vi "SetDev AFG Resource.vi"(8 "error in (no error)":errorcluster, 9 "AFG VISA Addr":refnum<visa-resource-name>, 10 "Simulated":bool, 11 "Actor_AFG in":refnum<class "Actor_AFG.lvclass">) -> (0 "error out":errorcluster, 3 "Actor_AFG out":refnum<class "Actor_AFG.lvclass">)   [LabVIEW 2020, in "Actor_AFG.lvlib" / "Actor_AFG.lvclass"]
uses:
  Actor_AFG.lvclass
  Actor_AFG.lvclass/Actor_AFG.ctl
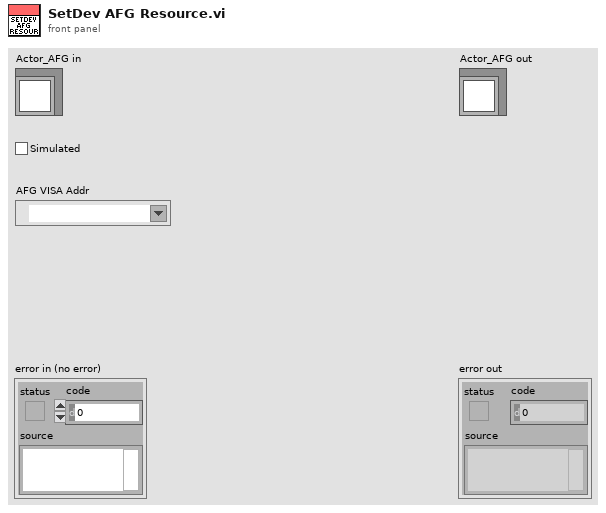
[diagram p1: front panel]
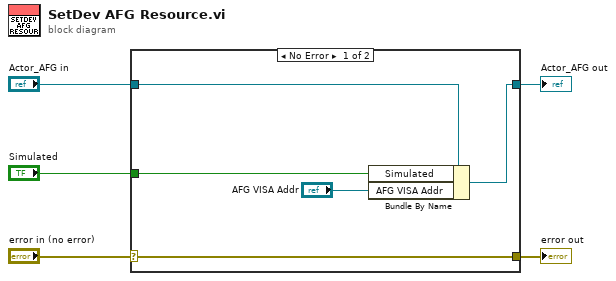
[diagram p0: block diagram]
diagram:
  n1 = case shown="No Error" "error in (no error)" {
    selector: "error in (no error)" -> [w10 w11]
    tunnel: [w10 w11] -> w4
    tunnel: [w8 w12] -> w2
    tunnel: "Actor_AFG in" -> [w9 w12]
    tunnel: "Simulated" -> [w7 _]
    frame No Error {
      n2 = Bundle By Name(cluster=w9, "Simulated"=w7, "AFG VISA Addr"="AFG VISA Addr") -> (w8:refnum<class "Actor_AFG.lvclass">)
    }
    frame Error {
    }
  }
  "error out" <- w4
  "Actor_AFG out" <- w2
